vi "ep_Hilbert Filter Design.vi"(8 "error in (no error)":errorcluster, 11 "fs":dbl) -> (0 "error out":errorcluster, 2 "Hilbert FIR filter":cluster{"h":dbl[], "delay":i32}, 3 "dup fs":dbl)   [LabVIEW 2014, in "NI_EP_Motor Monitoring.lvlib"]
uses:
  <vilib>/addons/Electrical Power/Motor Monitoring/NI_EP_Motor Monitoring.lvlib
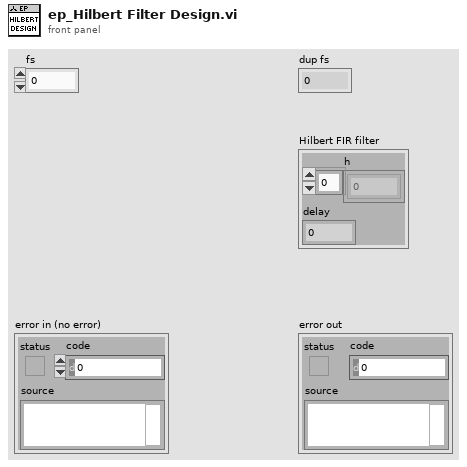
[diagram p1: front panel]
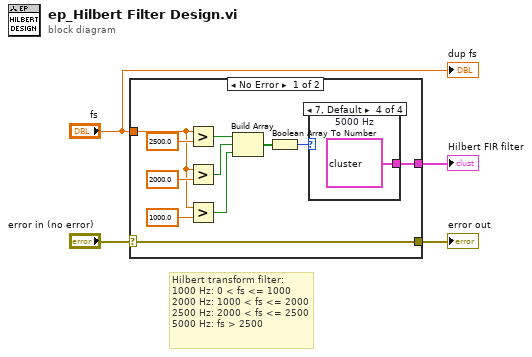
[diagram p0: block diagram]
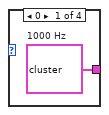
[diagram p2: hidden frame]
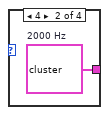
[diagram p3: hidden frame]
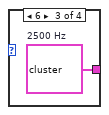
[diagram p4: hidden frame]
diagram:
  # "Hilbert transform filter:\n1000 Hz: 0 < fs <= 1000\n2000 Hz: 1000 < fs <= 2000\n2500 Hz: 2000 < fs <= 2500\n5000 Hz: fs > 2500"
  n1 = case shown="No Error" "error in (no error)" {
    selector: "error in (no error)" -> [w5 w20]
    tunnel: [w5 w20] -> w3
    tunnel: "fs" -> [w7 _]
    tunnel: [w6 _] -> w1
    frame No Error {
      n2 = Greater?(x=w7, y=2500.0) -> (0:w12:bool)
      n3 = Greater?(x=w7, y=2000.0) -> (0:w10:bool)
      n4 = Greater?(x=w7, y=1000.0) -> (0:w11:bool)
      n5 = Build Array(w12, w10, w11) -> (w9:bool[])
      n6 = Boolean Array To Number(Boolean array=w9) -> (number=w8:u32)
      n7 = case shown="7, Default" w8 {
        tunnel: [w16 w17 w18 w19] -> w6
        frame 0 {
          w16 = cluster{"h":dbl[], "delay":i32} {"h"=array[301 elements], "delay"=150}  # 1000 Hz
        }
        frame 4 {
          w17 = cluster{"h":dbl[], "delay":i32} {"h"=array[601 elements], "delay"=300}  # 2000 Hz
        }
        frame 6 {
          w18 = cluster{"h":dbl[], "delay":i32} {"h"=array[751 elements], "delay"=375}  # 2500 Hz
        }
        frame 7, Default {
          w19 = cluster{"h":dbl[], "delay":i32} {"h"=array[1501 elements], "delay"=750}  # 5000 Hz
        }
      }
    }
    frame Error {
    }
  }
  "error out" <- w3
  "Hilbert FIR filter" <- w1
  "dup fs" <- "fs"
